vi "From Serial Form.vi"(6 "Serial Version":T1, 10 "Deserializer in":refnum<class "Deserializer.lvclass">, 11 "U16 in":refnum<class "U16.lvclass">) -> (0 "error out":errorcluster, 2 "Deserializer out":refnum<class "Deserializer.lvclass">, 3 "U16 out":refnum<class "U16.lvclass">)   [LabVIEW 2014, in "Base Data Class.lvlib" / "U16.lvclass"]
uses:
  U16.lvclass
  <vilib>/NI/AQ Character Lineator/Deserializer/Deserializer.lvclass
  <vilib>/NI/AQ Character Lineator/Serialization Common/Serial Version.ctl
  U16.lvclass/U16.ctl
  <vilib>/NI/AQ Character Lineator/Serializable/Remove UInt16.vi
  Data.lvclass
  <vilib>/NI/AQ Character Lineator/Serializable/Serializable.lvclass
  <vilib>/NI/AQ Character Lineator/Serialization Common/Serialization Common.lvlib
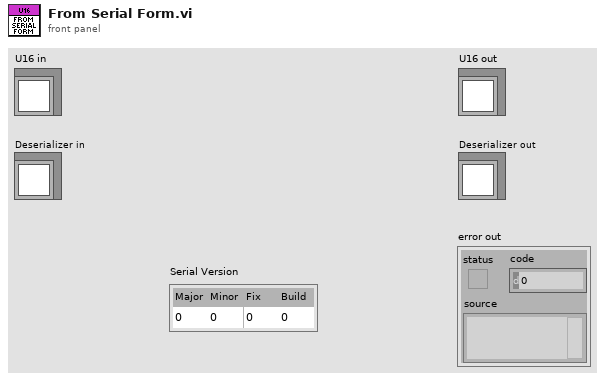
[diagram p1: front panel]
types:
  T1 = typedef "Serialization Common.lvlib/Serial Version.ctl" = cluster{"Major":u16, "Minor":u16, "Fix":u16, "Build":u16}
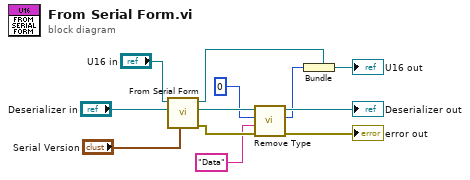
[diagram p0: block diagram]
diagram:
  n1 = call-parent "From Serial Form.vi"("Serial Version"="Serial Version", "Deserializer in"="Deserializer in", "Data in"="U16 in") -> ("error out"=w5:errorcluster, "Deserializer out"=w7:refnum<class "Deserializer.lvclass">, "Data out"=w3:refnum<class "U16.lvclass">)  [unwired: 6 in]
  n2 = call-poly <vilib>:"Remove Type.vi"("error in (no error)"=w5, "Name"="Data", "Default Value"=u16 0, "Deserializer in"=w7) -> ("error out"=→"error out":errorcluster, "Numeric"=w2:u16, "Deserializer out"=→"Deserializer out":refnum<class "Deserializer.lvclass">)  [unwired: 4 in, 1 out]
  n3 = Bundle(cluster=w3, w2) -> (→"U16 out":refnum<class "U16.lvclass">)
